vi "TempratureConversion.vi"() -> ()   [LabVIEW 2019]
uses:
  <vilib>/express/express arith-compare/Formula/XNode/ExpressFormulaBlockNode.xnode
panel:
  out "Kelvin":dbl(knob) scale=0.0..350.0
  out "Farenhit":dbl(knob) scale=0.0..250.0
  out "Kelvin":dbl(slide) scale=0.0..400.0
  out "Farenhit":dbl(slide) scale=0.0..300.0
  out "Kelvin":dbl
  out "Farenhit":dbl
  in  "Celsius":dbl
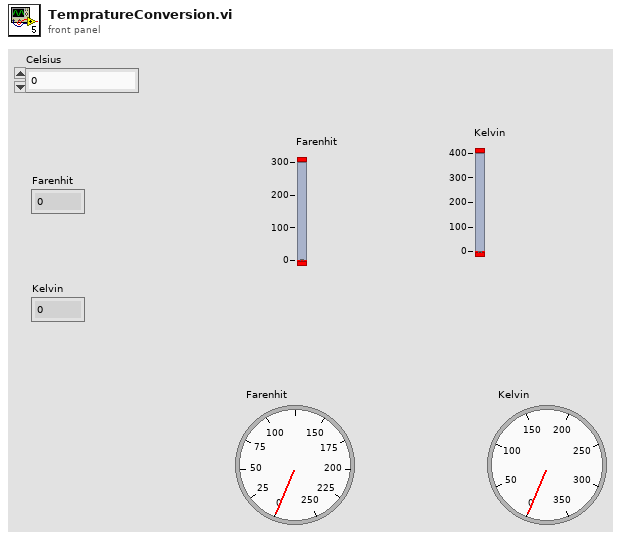
[diagram p1: front panel]
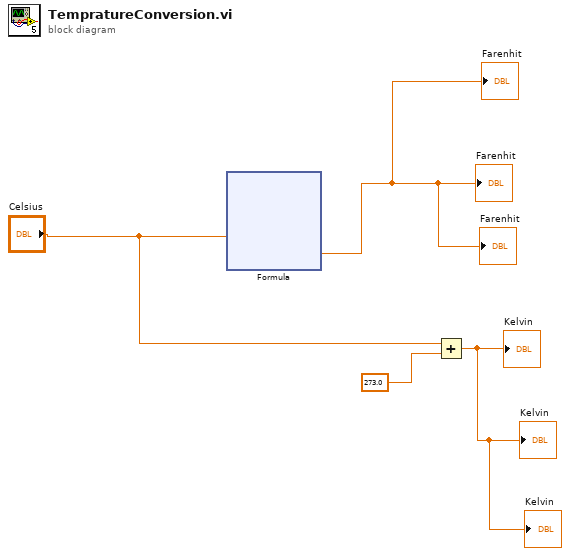
[diagram p0: block diagram]
diagram:
  n1 = xnode "Formula"("X1"="Celsius") -> ("Result"=→"Farenhit" →"Farenhit" →"Farenhit":dbl)  [unwired: 1 in, 1 out]
  n2 = Add(x="Celsius", y=273.0) -> (x+y=→"Kelvin" →"Kelvin" →"Kelvin":dbl)
